vi "DbaseCreateNewDialog.vi"(8 "error in (no error)":errorcluster, 11 "FAMM in":T3={"FAMM_PAQ_Layers"=0, "FAMM_PAQ_resolution"=0.0, "PAQ_TAGs"=[], "WAQ_TAGs"=[], "EAQ_TAGs"=[], "All_TAGs"=[], "PAQtagProps"=[], "WAQtagProps"=[], "EAQtagProps"=[], "DBAL_class"=refnum, "PAQ_memory"=[], "PAQupdates"=[], "FAMM_Size"={"other"=0, "1day"=0, "1week"=0}, "DatabaseFileExtention"="", "DatabaseSaveRate"=0.0, "Database_path"=path "G:/Sgraph_database", "DBAL-Queue"=refnum} {"FAMM_Size"."1week" format="%.0p"; "FAMM_Size"."1day" format="%.0p"; "FAMM_Size"."other" format="%.0p"; "EAQtagProps"."TagFunc" format="%08x"; "EAQtagProps"."RangeL" format="%.2f"; "EAQtagProps"."RangeH" format="%.2f"; "WAQtagProps"."TagFunc" format="%08x"; "WAQtagProps"."RangeL" format="%.2f"; "WAQtagProps"."RangeH" format="%.2f"; "PAQtagProps"."TagFunc" format="%08x"; "PAQtagProps"."RangeL" format="%.2f"; "PAQtagProps"."RangeH" format="%.2f"; "FAMM_PAQ_resolution" format="%.1p"}) -> (0 "error out":errorcluster, 3 "FAMM out":T3={"FAMM_PAQ_Layers"=0, "FAMM_PAQ_resolution"=0.0, "PAQ_TAGs"=[], "WAQ_TAGs"=[], "EAQ_TAGs"=[], "All_TAGs"=[], "PAQtagProps"=[], "WAQtagProps"=[], "EAQtagProps"=[], "DBAL_class"=refnum, "PAQ_memory"=[], "PAQupdates"=[], "FAMM_Size"={"other"=0, "1day"=0, "1week"=0}, "DatabaseFileExtention"="", "DatabaseSaveRate"=0.0, "Database_path"=path "G:/Sgraph_database", "DBAL-Queue"=refnum} {"FAMM_Size"."1week" format="%.0p"; "FAMM_Size"."1day" format="%.0p"; "FAMM_Size"."other" format="%.0p"; "EAQtagProps"."TagFunc" format="%08x"; "EAQtagProps"."RangeL" format="%.2f"; "EAQtagProps"."RangeH" format="%.2f"; "WAQtagProps"."TagFunc" format="%08x"; "WAQtagProps"."RangeL" format="%.2f"; "WAQtagProps"."RangeH" format="%.2f"; "PAQtagProps"."TagFunc" format="%08x"; "PAQtagProps"."RangeL" format="%.2f"; "PAQtagProps"."RangeH" format="%.2f"; "FAMM_PAQ_resolution" format="%.1p"})   [LabVIEW 2020, in "Sgraph_lib_V1.lvlib" / "FAMM.lvclass"]
doc: "Check if the database exists,\nIf yes and content is OK: then continue.\n\nIf parts are missing: Start user dialog and request what to do."
uses:
  FAMM.lvclass
  controls/FAMM-attributes.ctl
  Common/controls/typedef_com_TagProp.ctl
  DBAL/DBAL.lvclass
  PAQ-memory.lvclass
  DBAL/controls/DBAL_Command.ctl
  DBAL/controls/DBAL-commands.ctl
  controls/FAMM_DB_New_BIN_taginfo.ctl
  <vilib>/Utility/miscctls.llb/LVPointTypeDef.ctl
  HISW/controls/typedef_PAQsample.ctl
  HISW/HISW.lvclass
  Builds/Sgraph_lib_V1.lvlib
panel:
  out "sec SampleTime":dbl format="%#_2p"
  out "PAQ buffer":i32
  in  "PC memory usage":T1(radio)=enum."Item 2"
  in  "Cancel Button":bool
  in  "OK Button":bool
  in  "initial TAGs information":T2[](array[typedef]) {"Range L" format="%#_6p"; "Range H" format="%#_6p"}
  in  "Data Retention":T1(radio)
  in  "Database File Extention":string=".his"
  in  "Resolution":T1(radio)=enum."Item 1" caption="Periodic Samples (PAQ) Resolution"
  in  "Database type":enum32{"Item 0", "Item 1", "Item 2", "Item 3"}(radio)
  out "info":string
  # "TAG                  Units          Descrption                                                                      Range H    Range L"
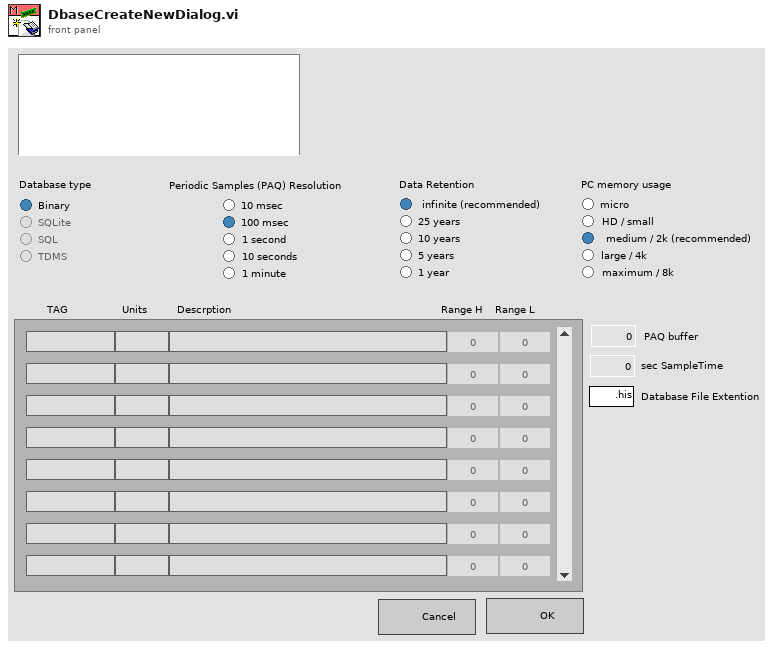
[diagram p1: front panel]
types:
  T1 = enum32{"Item 0", "Item 1", "Item 2", "Item 3", "Item 4"}
  T2 = typedef "Sgraph_lib_V1.lvlib/FAMM.lvclass/FAMM_DB_New_BIN_taginfo.ctl" = cluster{"TAG":string, "Units":string, "Description":string, "Range H":dbl, "Range L":dbl}
  T3 = typedef "Sgraph_lib_V1.lvlib/FAMM.lvclass/FAMM-attributes.ctl" = cluster{"FAMM_PAQ_Layers":i32, "FAMM_PAQ_resolution":dbl, "PAQ_TAGs":string[], "WAQ_TAGs":string[], "EAQ_TAGs":string[], "All_TAGs":string[], "PAQtagProps":T4[], "WAQtagProps":T4[], "EAQtagProps":T4[], "DBAL_class":refnum<data-value>, "PAQ_memory":refnum<data-value>[], "PAQupdates":timestamp[], "FAMM_Size":cluster{"other":i32, "1day":i32, "1week":i32}, "DatabaseFileExtention":string, "DatabaseSaveRate":dbl, "Database_path":path, "DBAL-Queue":refnum<queue>}
  T4 = typedef "Sgraph_lib_V1.lvlib/typedef_com_TagProp.ctl" = cluster{"Description":string, "EngUnits":string, "RangeH":dbl, "RangeL":dbl, "Resolution":i32, "Obsolete":bool, "ChangeDate":timestamp, "ChangeSource":string, "ChangeReason":string, "TagFunc":u32}
  T5 = typedef "LVPointTypeDef.ctl" = cluster{"Horizontal":i16, "Vertical":i16}
  T6 = typedef "typedef_PAQsample.ctl" = cluster{"Time Stamp":timestamp, "TAGs":string[], "status":u32[], "data":dbl[], "Source":string}
  T7 = cluster{"initial TAGs information":T2[], "Data Retention":enum32{"Item 0", "Item 1", "Item 2", "Item 3", "Item 4"}, "Database File Extention":string, "PC memory usage":enum32{"Item 0", "Item 1", "Item 2", "Item 3", "Item 4"}, "Resolution":enum32{"Item 0", "Item 1", "Item 2", "Item 3", "Item 4"}}
  T8 = typedef "typedef-DAQ-datagram.ctl" = cluster{"Time Stamp":timestamp, "Source":string, "Data":variant, "Qtype":T9}
  T9 = typedef "typedef-Qtype.ctl" = enum16{"PAQ", "WAQ", "EAQ", "End-Service"}
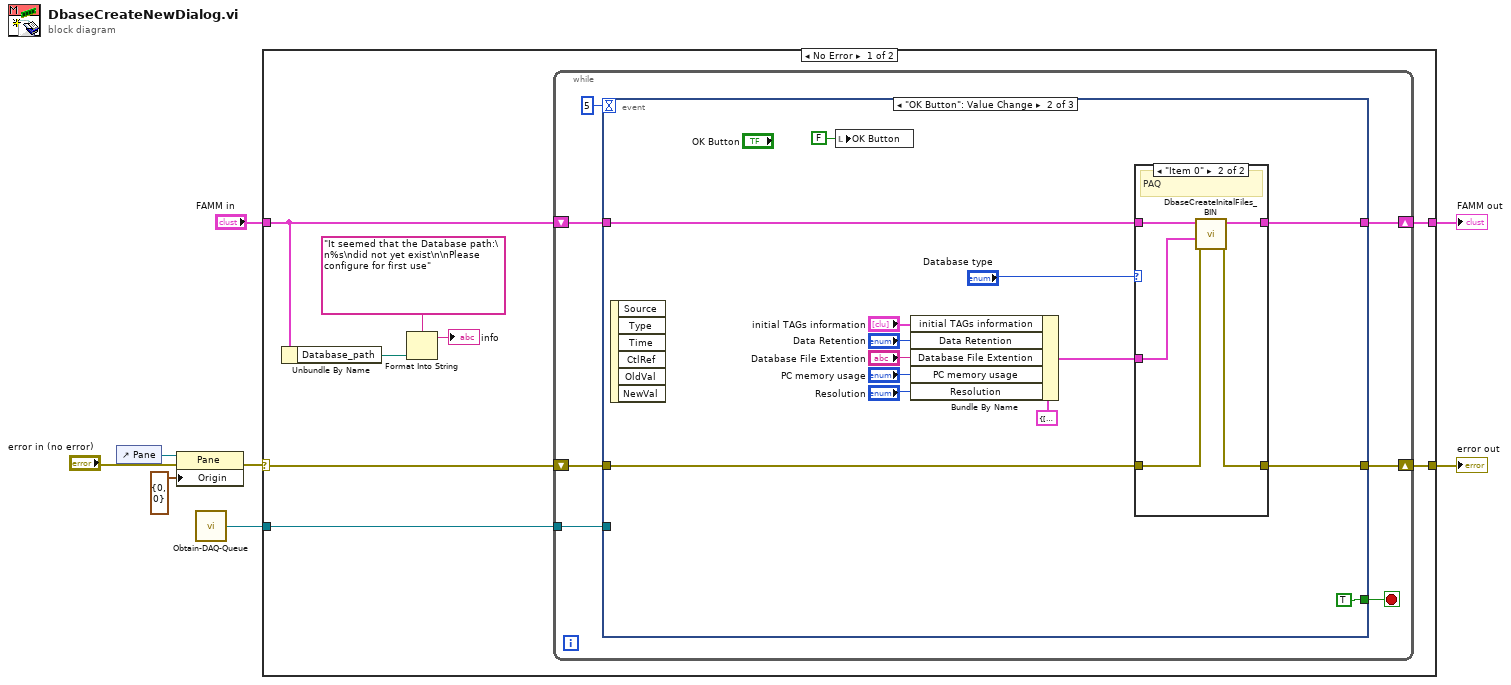
[diagram p0: block diagram]
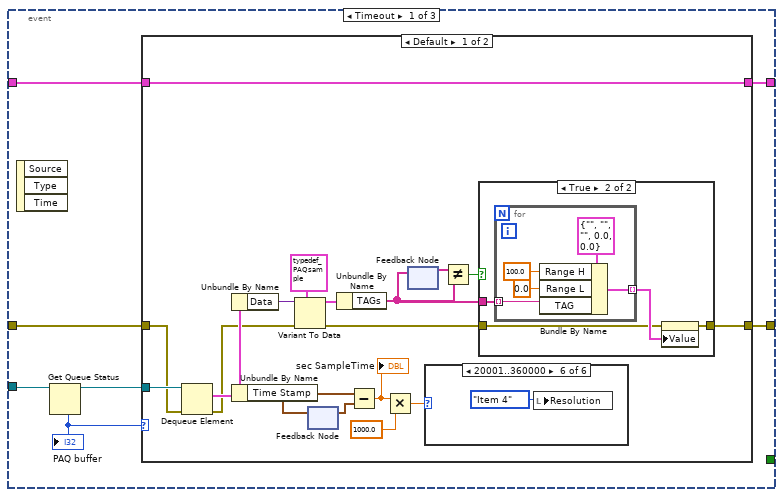
[diagram p2: hidden frame]
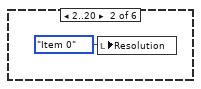
[diagram p5: hidden frame]
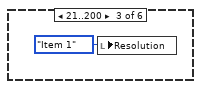
[diagram p6: hidden frame]
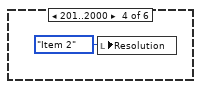
[diagram p7: hidden frame]
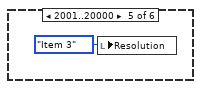
[diagram p8: hidden frame]
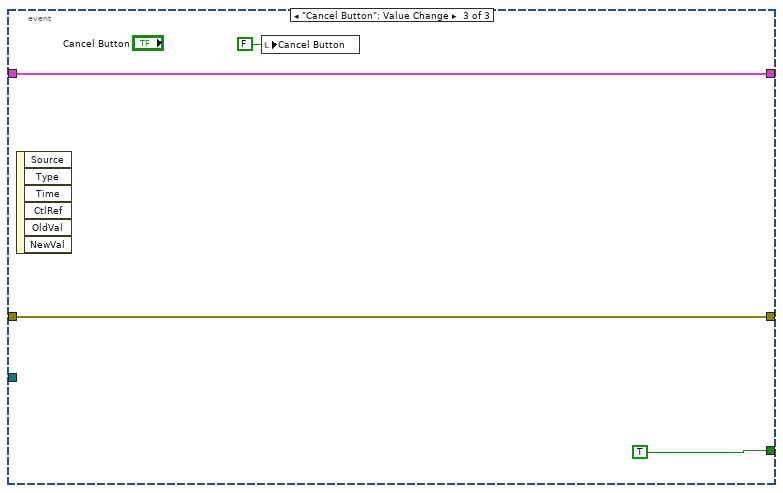
[diagram p11: hidden frame]
diagram:
  n1 = control-ref of="Pane"() -> (w5:refnum<vi>)
  n2 = property class="Pane"(reference=w5, error in="error in (no error)", "Origin"=T5 {"Horizontal"=0, "Vertical"=0}) -> (error out=w3:errorcluster)  [unwired: 1 out]
  n3 = call "Obtain-DAQ-Queue.vi"() -> ("DAQ-Queue"=w1:refnum<queue>)  [unwired: 7 in]
  n4 = case shown="No Error" w3 {
    selector: w3 -> [w13 w92]
    tunnel: [w11 w92] -> w8
    tunnel: [w10 w91] -> w6
    tunnel: "FAMM in" -> [w12 w91]
    tunnel: w1 -> [w9 _]
    frame No Error {
      n5 = Unbundle By Name(w12) -> ("Database_path"=w16:path)
      n6 = Format Into String(format string="It seemed that the Database path:\n%s\ndid not yet exist\n\nPlease configure for first use", w16) -> (resulting string=→"info":string)  [unwired: 2 in, 1 out]
      n7 = while {
        shift-right: [w19] -> w11
        shift-left: w13 -> [w21]
        shift-right: [w20] -> w10
        shift-left: w12 -> [w22]
        tunnel: w9 -> [w17]
        stop <- w18 stop-if-true
        n8 = event shown="[1] \"OK Button\": Value Change" {
          selector: _ -> [_ _ _]
          dyn-events: _ -> [_ _ _]
          timeout: 5 -> [_ _ _]
          tunnel: w22 -> [w28 w76 w89]
          tunnel: w21 -> [w27 w75 w88]
          tunnel: [w26 w73 w89] -> w20
          tunnel: [w25 w74 w88] -> w19
          tunnel: [_ TRUE TRUE] -> w18
          tunnel: w17 -> [w30 _ _]
          event Timeout {
            n9 = event-data() -> ()  [unwired: 1 in, 3 out]
            n10 = Get Queue Status(queue=w30) -> (queue out=w24:refnum<queue>, # elements in queue=w29:i32)  [unwired: 2 in, 6 out]
            "PAQ buffer" <- w29
            n11 = case shown="Default" w29 {
              tunnel: w28 -> [w48 w65]
              tunnel: w27 -> [w46 w64]
              tunnel: [w48 w65] -> w26
              tunnel: [w31 w64] -> w25
              tunnel: w24 -> [w47 _]
              frame Default {
                n12 = Dequeue Element(queue=w47, error in (no error)=w46) -> (element=w40:T8, error out=w33:errorcluster)  [unwired: 1 in, 2 out]
                n13 = Unbundle By Name(w40) -> ("Data"=w34:variant)
                n14 = Unbundle By Name(w40) -> ("Time Stamp"=w45:timestamp)
                n15 = Variant To Data(error in=w33, type=T6 {"Time Stamp"=timestamp(0 s since 1904-01-01), "TAGs"=[], "status"=[], "data"=[], "Source"="DAQ"} ("PAQ IN"), Variant=w34) -> (data=w38:T6, error out=w32:errorcluster)
                n16 = feedback-in #1(w45) -> ()
                n17 = feedback #1() -> (w44:timestamp)  [unwired: 1 in]
                n18 = Unbundle By Name(w38) -> ("TAGs"=w35:string[])
                n19 = Subtract(x=w45, y=w44) -> (x-y=w43:dbl)
                "sec SampleTime" <- w43
                n20 = Multiply(x=w43, y=1000.0) -> (x*y=w41:dbl)
                n21 = feedback #2() -> (w37:string[])  [unwired: 1 in]
                n22 = feedback-in #2(w35) -> ()
                n23 = case shown="20001..360000" w41 {
                  frame Default {
                  }
                  frame 2..20 {
                    n24 = local write "Resolution"(T1."Item 0" ("Period")) -> ()
                  }
                  frame 21..200 {
                    n25 = local write "Resolution"(T1."Item 1" ("Period")) -> ()
                  }
                  frame 201..2000 {
                    n26 = local write "Resolution"(T1."Item 2" ("Period")) -> ()
                  }
                  frame 2001..20000 {
                    n27 = local write "Resolution"(T1."Item 3" ("Period")) -> ()
                  }
                  frame 20001..360000 {
                    n28 = local write "Resolution"(T1."Item 4" ("Period")) -> ()
                  }
                }
                n29 = Not Equal?(x=w37, y=w35) -> (x != y?=w36:bool)
                n30 = case shown="True" w36 {
                  tunnel: w35 -> [_ w53]
                  tunnel: w32 -> [w49 w51]
                  tunnel: [w49 w50] -> w31
                  frame False {
                  }
                  frame True {
                    n31 = for {
                      tunnel: w53 -> [w57] mode=indexing
                      tunnel: [w54] -> w52 mode=indexing
                      n32 = Bundle By Name(cluster=T2 {"TAG"="", "Units"="", "Description"="", "Range H"=0.0, "Range L"=0.0} ("TAGinfo"), "Range H"=100.0, "Range L"=0.0, "TAG"=w57) -> (w54:T2)
                    }
                    n33 = property on="initial TAGs information" class="Arr (strict)"(error in=w51, "Value"=w52) -> (error out=w50:errorcluster)  [unwired: 1 in, 1 out]
                  }
                }
              }
              frame 0 {
              }
            }
          }
          event "OK Button": Value Change {
            n34 = event-data() -> ()  [unwired: 1 in, 6 out]
            n35 = local write "OK Button"(FALSE ("OK Button")) -> ()
            n36 = Bundle By Name(cluster=T7 {"initial TAGs information"=[{"TAG"="ch0001", "Units"="ºC", "Description"="", "Range H"=100.0, "Range L"=0.0}, {"TAG"="ch0002", "Units"="ºC", "Description"="", "Range H"=100.0, "Range L"=0.0}, {"TAG"="ch0003", "Units"="ºC", "Description"="", "Range H"=100.0, "Range L"=0.0}, {"TAG"="ch0004", "Units"="ºC", "Description"="", "Range H"=100.0, "Range L"=0.0}, {"TAG"="ch0005", "Units"="ºC", "Description"="", "Range H"=100.0, "Range L"=0.0}, {"TAG"="ch0006", "Units"="ºC", "Description"="", "Range H"=100.0, "Range L"=0.0}, {"TAG"="ch0007", "Units"="ºC", "Description"="", "Range H"=100.0, "Range L"=0.0}, {"TAG"="ch0008", "Units"="ºC", "Description"="", "Range H"=100.0, "Range L"=0.0}, {"TAG"="ch0009", "Units"="ºC", "Description"="", "Range H"=100.0, "Range L"=0.0}, {"TAG"="ch0010", "Units"="ºC", "Description"="", "Range H"=100.0, "Range L"=0.0}], "Data Retention"=enum."Item 0", "Database File Extention"=".his", "PC memory usage"=enum."Item 2", "Resolution"=enum."Item 0"}, "initial TAGs information"="initial TAGs information", "Data Retention"="Data Retention", "Database File Extention"="Database File Extention", "PC memory usage"="PC memory usage", "Resolution"="Resolution") -> (w66:T7)
            n37 = case shown="\"Item 0\"" "Database type" {
              tunnel: w76 -> [w81 w85]
              tunnel: w75 -> [w80 w83]
              tunnel: [w80 w84] -> w74
              tunnel: [w81 w86] -> w73
              tunnel: w66 -> [_ w82]
              frame Default {
              }
              frame "Item 0" {
                # "PAQ"
                n38 = call "DbaseCreateInitalFiles_BIN.vi"("error in (no error)"=w83, "DB_SetupData"=w82, "FAMM in"=w85) -> ("error out"=w84:errorcluster, "FAMM out"=w86:T3)  [unwired: 7 in]
              }
            }
          }
          event "Cancel Button": Value Change {
            n39 = event-data() -> ()  [unwired: 1 in, 6 out]
            n40 = local write "Cancel Button"(FALSE ("Cancel Button")) -> ()
          }
        }
      }
    }
    frame Error {
    }
  }
  "error out" <- w8
  "FAMM out" <- w6
